vi "Dequeue Broadcast Message by Message.vi"(8 "error in (no error)":errorcluster, 9 "Timeout (-1)":i32=-1, 10 "Message":string, 11 "Event Registration Refnum":refnum<event-registration>) -> (0 "error out":errorcluster, 1 "Message Data":variant, 2 "Message":string, 3 "Event Registration Refnum Out":refnum<event-registration>, 4 "Timed Out?":bool)   [LabVIEW 2020, in "Broadcast Event Dequeuers.lvlib"]
doc: "Dequeue Broadcast messages filtering by message. The time out for this VI has an error margin of up to one time-out period in edge cases."
uses:
  Broadcast Event Dequeuers.lvlib
  Process/Protected/Broadcasting/Broadcast Message Cluster.ctl
  Process/Process.lvclass
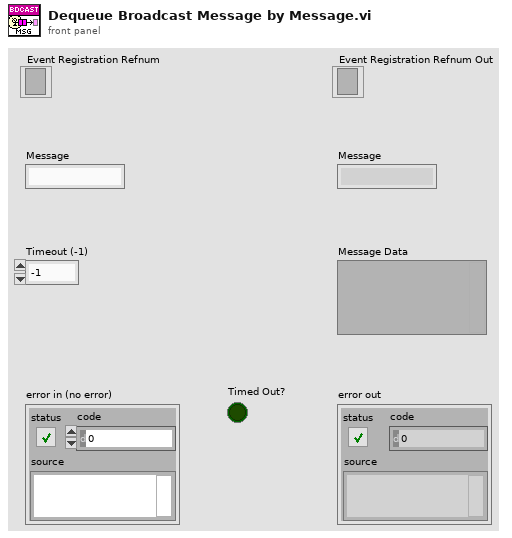
[diagram p1: front panel]
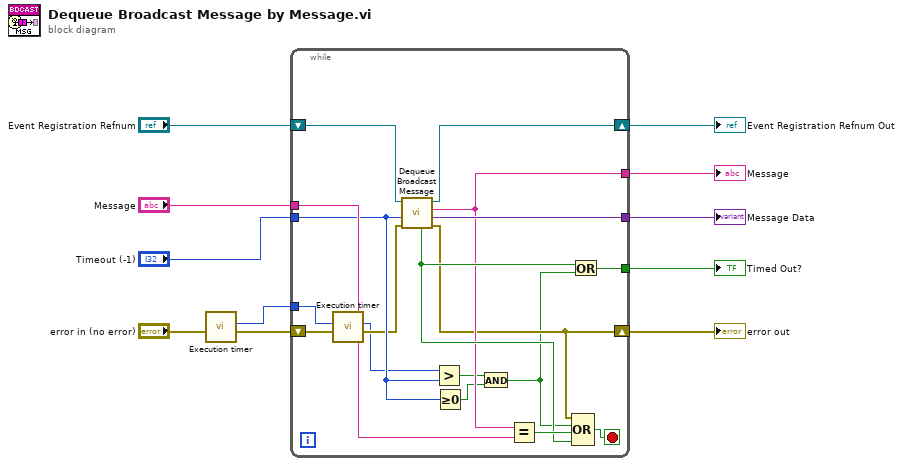
[diagram p0: block diagram]
diagram:
  n1 = call "Execution timer.vi"("error in (no error)"="error in (no error)") -> ("error out"=w2:errorcluster, "Current or Duration [ms]"=w1:u32)  [unwired: 9 in]
  n2 = while {
    tunnel: [w21] -> w7
    tunnel: [w26] -> w6
    tunnel: [w13] -> w5
    tunnel: "Timeout (-1)" -> [w18]
    shift-right: [w28] -> w10
    shift-left: "Event Registration Refnum" -> [w29]
    shift-right: [w14] -> w8
    shift-left: w2 -> [w27]
    tunnel: "Message" -> [w25]
    tunnel: w1 -> [w16]
    stop <- w23 stop-if-true
    n3 = call "Execution timer.vi"("error in (no error)"=w27, "millisecond timer value"=w16) -> ("error out"=w17:errorcluster, "Current or Duration [ms]"=w15:u32)  [unwired: 8 in]
    n4 = call "Dequeue Broadcast Message.vi"("error in (no error)"=w17, "Timeout (-1)"=w18, "Event Registration Refnum"=w29) -> ("error out"=w14:errorcluster, "Message Data"=w26:variant, "Message"=w21:string, "Event Registration Refnum Out"=w28:refnum<event-registration>, "Timed Out?"=w22:bool)  [unwired: 3 in, 1 out]
    n5 = Greater?(x=w15, y=w18) -> (0:w20:bool)
    n6 = Greater Or Equal To 0?(x=w18) -> (x >= 0?=w19:bool)
    n7 = And(x=w20, y=w19) -> (x .and. y?=w12:bool)
    n8 = Equal?(x=w21, y=w25) -> (x = y?=w24:bool)
    n9 = Or(x=w22, y=w12) -> (x .or. y?=w13:bool)
    n10 = Compound Arithmetic op=OR(w14, w12, w24, w22) -> (w23:bool)
  }
  "Event Registration Refnum Out" <- w10
  "Message Data" <- w6
  "Message" <- w7
  "error out" <- w8
  "Timed Out?" <- w5
